vi "Demo HttpServer.vi"() -> ()   [LabVIEW 2021, in "HttpServer.lvlib"]
uses:
  HttpServer.lvlib
  <vilib>/Utility/error.llb/Error Cluster From Error Code.vi
  SubVIs/Page.vit
  <vilib>/ErrorRing/Error Ring.xnode
panel:
  out "Http Server":string
  out "ms Elapsed":u32
  in  "Stop":bool
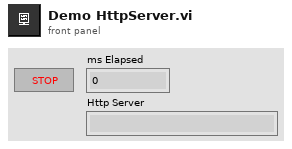
[diagram p1: front panel]
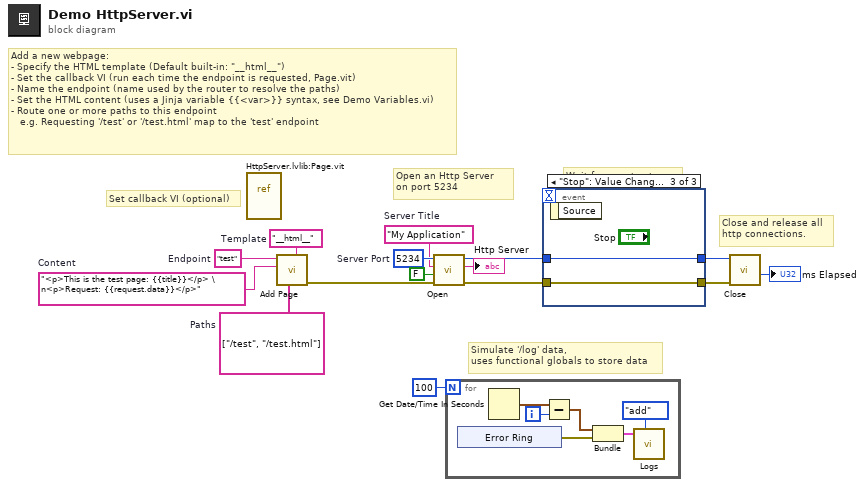
[diagram p0: block diagram]
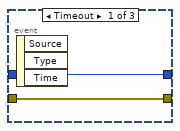
[diagram p2: hidden frame]
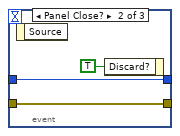
[diagram p3: hidden frame]
diagram:
  w7 = "My Application"  # Server Title
  w10 = u16 5234  # Server Port
  w12 = string[] ["/test", "/test.html"]  # Paths
  w13 = "__html__"  # Template
  w14 = "<p>This is the test page: {{title}}</p> \n<p>Request: {{request.data}}</p>"  # Content
  w15 = "test"  # Endpoint
  # "Close and release all\nhttp connections."
  # "Wait for user to stop"
  # "Open an Http Server\non port 5234"
  # "Add a new webpage:\n- Specify the HTML template (Default built-in: \"__html__\")\n- Set the callback VI (run each time the endpoint is requested, Page.vit)\n- Name the endpoint (name used by the router to resolve the paths)\n- Set the HTML content (uses a Jinja variable {{<var>}} syntax, see Demo Variables.vi)\n- Route one or more paths to this endpoint\n   e.g. Requesting '/test' or '/test.html' map to the 'test' endpoint"
  # "Simulate '/log' data,\nuses functional globals to store data"
  # "Set callback VI (optional)"
  n1 = vi-ref "HttpServer.lvlib:Page.vit"() -> ()  [unwired: 1 out]
  n2 = call "Add Page.vi"("Template (\"\")"=w13, "Paths"=w12, "Content"=w14, "Endpoint"=w15) -> ("error out"=w5:errorcluster)  [unwired: 7 in]
  n3 = call "Open.vi"("error in (no error)"=w5, "Open FP? (F)"=FALSE, "Server Title"=w7, "Server Port in"=w10) -> ("error out"=w1:errorcluster, "Http Server"=→"Http Server":string, "Server Port out"=w3:u16)  [unwired: 5 in]
  n4 = for {
    N: 100 -> [_]
    i -> [w18]
    n5 = xnode "Error Ring"() -> ("error out"=w20:errorcluster)
    n6 = Get Date/Time In Seconds() -> (seconds since 1Jan1904=w17:timestamp)
    n7 = Subtract(x=w17, y=w18) -> (x-y=w16:timestamp)
    n8 = Bundle(w16, "error out"=w20) -> (w19:cluster{timestamp, "error out":errorcluster})  [unwired: 1 in]
    n9 = call "Logs.vi"("Action"=enum8{"noop", "add", "clear"}."add", "log"=w19) -> ()  [unwired: 9 in, 1 out]
  }
  n10 = event shown="[2] \"Stop\": Value Change" {
    selector: _ -> [_ _ _]
    dyn-events: _ -> [_ _ _]
    timeout: _ -> [_ _ _]
    tunnel: [w27 w29 w32] -> w4
    tunnel: w3 -> [w27 w29 w32]
    tunnel: [w26 w28 w31] -> w2
    tunnel: w1 -> [w26 w28 w31]
    event Timeout {
      n11 = event-data() -> ()  [unwired: 1 in, 3 out]
    }
    event Panel Close? {
      n12 = event-data() -> ()  [unwired: 1 in, 1 out]
      n13 = event-data("Discard?"=TRUE) -> ()  [unwired: 1 in, 1 out]
    }
    event "Stop": Value Change {
      n14 = event-data() -> ()  [unwired: 1 in, 1 out]
    }
  }
  n15 = call "Close.vi"("error in (no error)"=w2, "Server Port in"=w4) -> ("ms Elapsed"=→"ms Elapsed":u32)  [unwired: 8 in, 1 out]
